vi "tcs shm put Sample kernel Site LV.vi"(8 "error in (no error)":errorcluster, 11 "kernel_Site_Ctl":T1) -> (0 "error out":errorcluster, 2 "function return":i32, 3 "kernel_Site_Ctl out":T1)   [LabVIEW 2016, in "SALLV_tcs.lvlib"]
doc: "int tcs_shm_putSample_kernel_SiteLV(tcs_kernel_SiteLV *kernel_Site_Ctl );"
uses:
  SALLV_tcs.lvlib
  SALLV_tcs.so
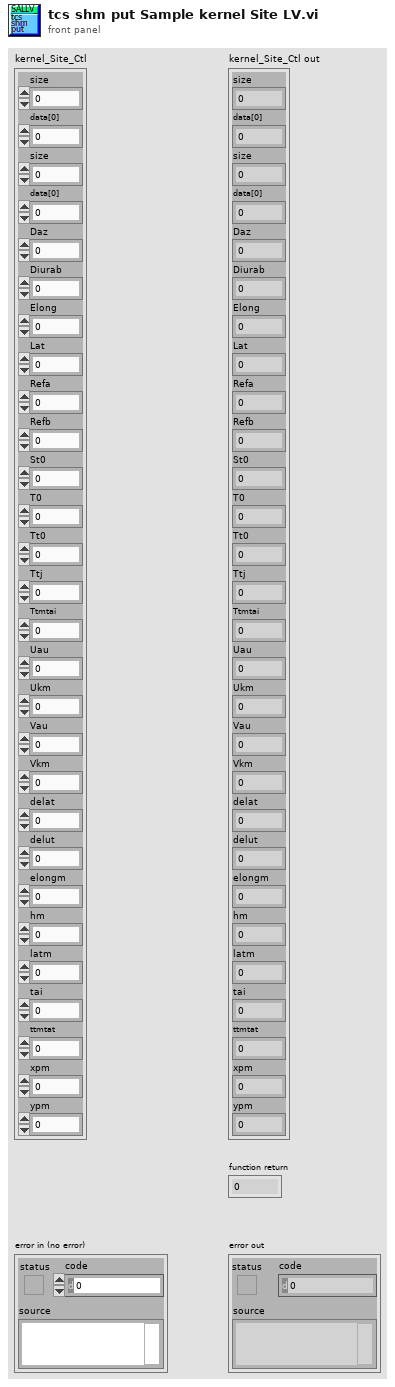
[diagram p1: front panel]
types:
  T1 = cluster{"size":i32, "data[0]":sgl, "size":i32, "data[0]":sgl, "Daz":sgl, "Diurab":sgl, "Elong":sgl, "Lat":sgl, "Refa":sgl, "Refb":sgl, "St0":sgl, "T0":sgl, "Tt0":sgl, "Ttj":sgl, "Ttmtai":sgl, "Uau":sgl, "Ukm":sgl, "Vau":sgl, "Vkm":sgl, "delat":sgl, "delut":sgl, "elongm":sgl, "hm":sgl, "latm":sgl, "tai":sgl, "ttmtat":sgl, "xpm":sgl, "ypm":sgl}
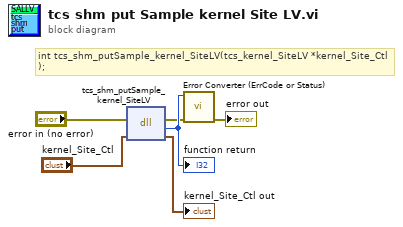
[diagram p0: block diagram]
diagram:
  # "int tcs_shm_putSample_kernel_SiteLV(tcs_kernel_SiteLV *kernel_Site_Ctl );"
  n1 = dll-call lib="home/andres/Desktop/SALLV_tcs/SALLV_tcs.*" fn="tcs_shm_putSample_kernel_SiteLV"(error in="error in (no error)", "kernel_Site_Ctl"="kernel_Site_Ctl") -> (error out=w2:errorcluster, w6:i32, "kernel_Site_Ctl"=→"kernel_Site_Ctl out":T1)  [unwired: 2 in, 1 out]
  "function return" <- w6
  n2 = call "Error Converter (ErrCode or Status).vi"("error in (no error)"=w2, "error code"=w6) -> ("error out"=→"error out":errorcluster)  [unwired: 9 in]
